vi "Factory.vi"(10 "Blacklist Class":T1, 11 "VI Refnum":refnum<vi>) -> (0 "error out":errorcluster, 3 "Blacklist out":refnum<class "Blacklist.lvclass">)   [LabVIEW 2014, in "BuildSecurity.lvlib" / "Blacklist.lvclass"]
doc: "Factory to create the correct blacklist processor based on the provided class."
uses:
  Blacklist.lvclass
  BlacklistClassInfo.ctl
  Blacklist.lvclass/Blacklist.ctl
  BuildSecurity.lvlib
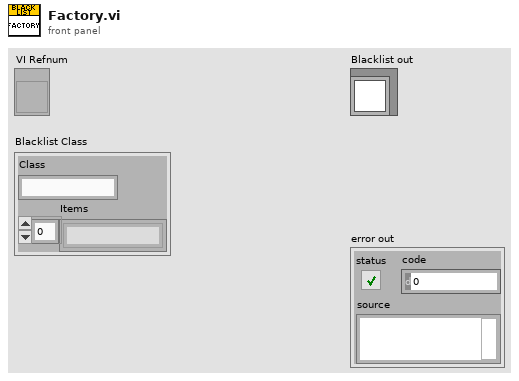
[diagram p1: front panel]
types:
  T1 = typedef "BuildSecurity.lvlib/BlacklistClassInfo.ctl" = cluster{"Class":string, "Items":string[]}
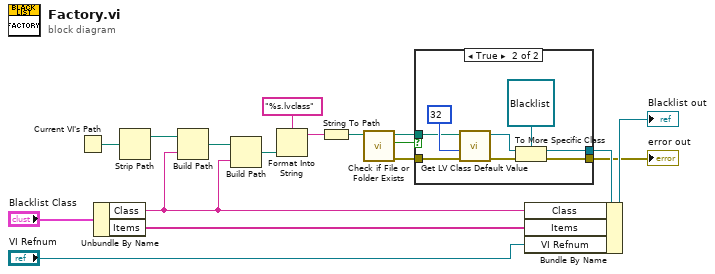
[diagram p0: block diagram]
diagram:
  n1 = Current VI's Path() -> (path=w11:path)
  n2 = Unbundle By Name("Blacklist Class") -> ("Class"=w5:string, "Items"=w4:string[])
  n3 = Strip Path(path=w11) -> (stripped path=w10:path)  [unwired: 1 out]
  n4 = Build Path(base path=w10, name or relative path=w5) -> (appended path=w13:path)
  n5 = Build Path(base path=w13, name or relative path=w5) -> (appended path=w12:path)
  n6 = Format Into String(format string="%s.lvclass", w12) -> (resulting string=w15:string)  [unwired: 2 in, 1 out]
  n7 = String To Path(string=w15) -> (path=w14:path)
  n8 = call <vilib>:"Check if File or Folder Exists.vi"("path"=w14) -> ("error out"=w8:errorcluster, "file or folder exists?"=w9:bool, "dup path"=w7:path)  [unwired: 8 in]
  n9 = case shown="True" w9 {
    tunnel: w8 -> [w18 w25]
    tunnel: w7 -> [_ w24]
    tunnel: [w18 w20] -> w1
    tunnel: [_ w19] -> w6
    frame False {
    }
    frame True {
      n10 = call <vilib>:"Get LV Class Default Value.vi"("error in (no error)"=w25, "options"=u32 32, "class path"=w24) -> ("error out"=w23:errorcluster, "object"=w22:refnum<class>)  [unwired: 7 in]
      n11 = To More Specific Class(target class=refnum<class "Blacklist.lvclass"> refnum ("Blacklist out"), reference=w22, error in=w23) -> (specific class reference=w19:refnum<class "Blacklist.lvclass">, error out=w20:errorcluster)
    }
  }
  "error out" <- w1
  n12 = Bundle By Name(cluster=w6, "Class"=w5, "Items"=w4, "VI Refnum"="VI Refnum") -> (→"Blacklist out":refnum<class "Blacklist.lvclass">)
